vi "DAQNavi Write (Analog 2D U32 NChan NSamp).vi"(8 "error in (no error)":errorcluster, 9 "timeout":dbl=10.0, 10 "data":u32[][](array[numeric]), 11 "task in":i32) -> (0 "error out":errorcluster, 2 "number of samples written per channel":u32, 3 "task out":i32)   [LabVIEW 2020]
uses:
  DAQNavi_LV.dll
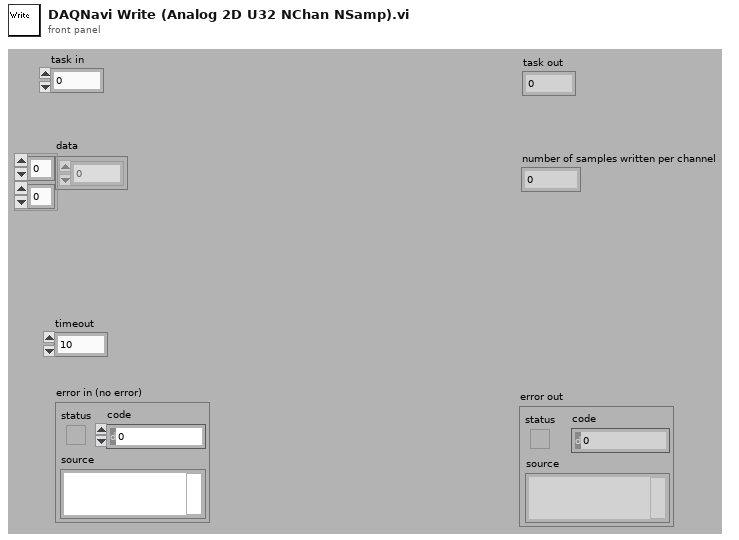
[diagram p1: front panel]
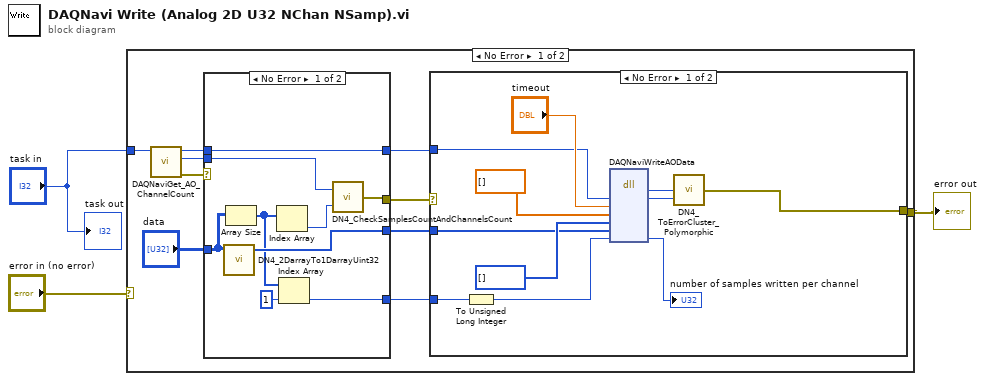
[diagram p0: block diagram]
diagram:
  n1 = case shown="No Error" "error in (no error)" {
    selector: "error in (no error)" -> [_ w37]
    tunnel: [w9 w37] -> w2
    tunnel: "task in" -> [w10 _]
    frame No Error {
      n2 = call "DAQNaviGet_AO_ChannelCount.vi"("task in"=w10) -> ("error out"=w13:errorcluster, "channel count"=w12:i32, "task out"=w11:i32)  [unwired: 1 in, 7 out]
      n3 = case shown="No Error" w13 {
        selector: w13 -> [_ w24]
        tunnel: w12 -> [w21 _]
        tunnel: [w20 w24] -> w7
        tunnel: [w22 w23] -> w8
        tunnel: w11 -> [w22 w23]
        tunnel: "data" -> [w19 _]
        tunnel: [w18 _] -> w5
        tunnel: [w14 _] -> w4
        frame No Error {
          n4 = call "DN4_2DarrayTo1DarrayUint32.vi"("2Darray"=w19) -> ("1Darray"=w18:u32[])  [unwired: 5 out]
          n5 = Array Size(array=w19) -> (size(s)=w16:i32[])
          n6 = Index Array(array=w16) -> (element=w17:i32)  [unwired: 1 in]
          n7 = Index Array(array=w16, index=1) -> (element=w14:i32)
          n8 = call "DN4_CheckSamplesCountAndChannelsCount.vi"("samples count"=w17, "channel count"=w21) -> ("error out"=w20:errorcluster)
        }
        frame Error {
        }
      }
      n9 = case shown="No Error" w7 {
        selector: w7 -> [_ w36]
        tunnel: [w35 w36] -> w9
        tunnel: w8 -> [w31 _]
        tunnel: w5 -> [w26 _]
        tunnel: w4 -> [w30 _]
        frame No Error {
          n10 = To Unsigned Long Integer(number=w30) -> (unsigned 32bit integer=w29:u32)
          n11 = dll-call lib="DAQNavi_LV.dll" fn="DAQNaviWriteAOData"("taskID"=w31, "timeout"="timeout", "scaledData"=dbl[] [], "rawData16"=u16[] [] ("rawData32"), "rawData32"=w26, "samples"=w29) -> ("return type"=w32:i32, "taskID"=w25:i32, "samples"=→"number of samples written per channel":u32)  [unwired: 5 in, 4 out]
          n12 = call "DN4_ToErrorCluster_Polymorphic.vi"("task id"=w25, "error code"=w32) -> ("error out"=w35:errorcluster)  [unwired: 3 out]
        }
        frame Error {
        }
      }
    }
    frame Error {
    }
  }
  "error out" <- w2
  "task out" <- "task in"
